vi "4 Bits Write.vi"(6 "E?E1:E2 (E1)":bool=TRUE, 9 "RS":bool, 10 "LCD data/cmd":u8 format="%.0x", 11 "device connection map":T1={"RS"="RS", "R/W"="RW", "E1"="E1", "E2"="E2", "DB4"="DB4", "DB5"="DB5", "DB6"="DB6", "DB7"="DB7"}) -> ()   [LabVIEW 2017, in "HD44780 FPGA.lvlib"]
uses:
  HD44780 FPGA.lvlib
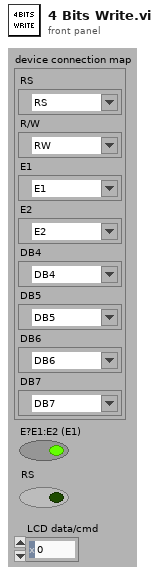
[diagram p1: front panel]
types:
  T1 = cluster{"RS":refnum<k21>, "R/W":refnum<k21>, "E1":refnum<k21>, "E2":refnum<k21>, "DB4":refnum<k21>, "DB5":refnum<k21>, "DB6":refnum<k21>, "DB7":refnum<k21>}
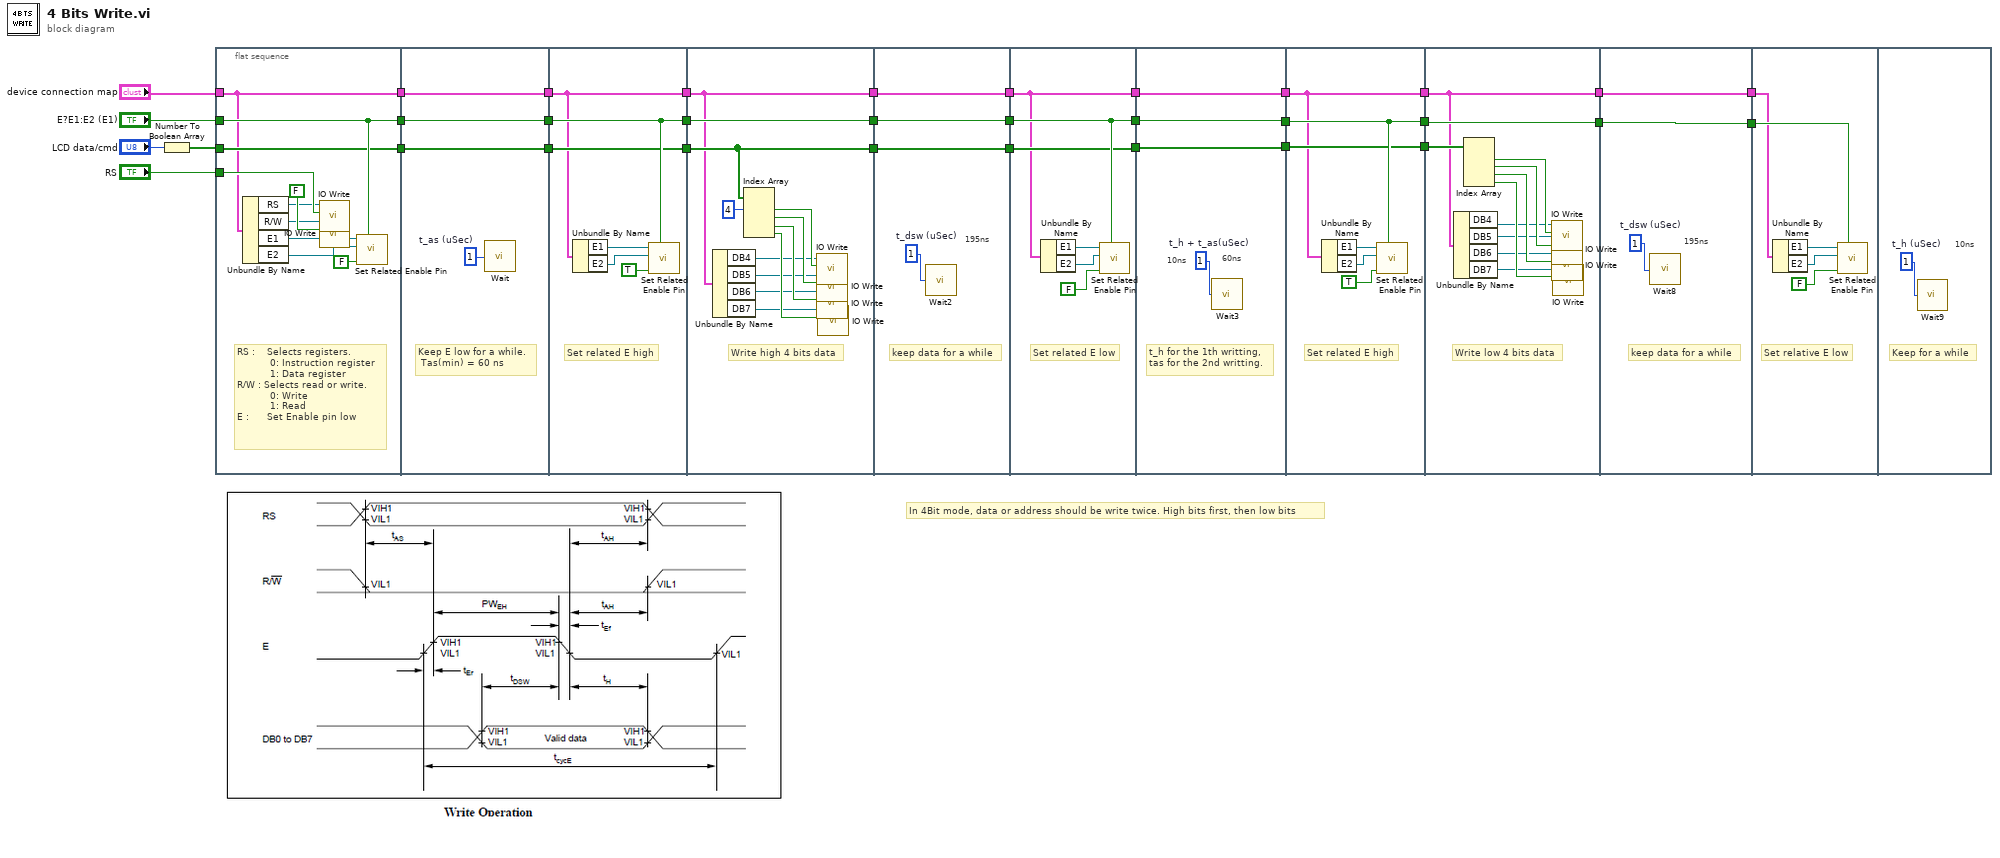
[diagram p0: block diagram]
diagram:
  # "In 4Bit mode, data or address should be write twice. High bits first, then low bits"
  n1 = Number To Boolean Array(number="LCD data/cmd") -> (Boolean array=w32:bool[])
  n2 = flat-sequence {
    tunnel: [w39] -> w29
    tunnel: [w40] -> w28
    tunnel: [w34] -> w11
    tunnel: w32 -> [w39]
    tunnel: "RS" -> [w43]
    tunnel: "E?E1:E2 (E1)" -> [w40]
    tunnel: "device connection map" -> [w34]
    tunnel: w29 -> [w46]
    tunnel: [w46] -> w27
    tunnel: w28 -> [w45]
    tunnel: [w45] -> w26
    tunnel: [w44] -> w12
    tunnel: w11 -> [w44]
    tunnel: w27 -> [w51]
    tunnel: [w51] -> w25
    tunnel: w26 -> [w52]
    tunnel: [w52] -> w24
    tunnel: [w48] -> w13
    tunnel: w12 -> [w48]
    tunnel: w25 -> [w64]
    tunnel: [w64] -> w23
    tunnel: w24 -> [w59]
    tunnel: [w59] -> w22
    tunnel: w13 -> [w54]
    tunnel: [w54] -> w8
    tunnel: w23 -> [w68]
    tunnel: [w68] -> w21
    tunnel: w22 -> [w67]
    tunnel: [w67] -> w20
    tunnel: [w66] -> w9
    tunnel: w8 -> [w66]
    tunnel: w21 -> [w73]
    tunnel: [w73] -> w19
    tunnel: w20 -> [w75]
    tunnel: [w75] -> w18
    tunnel: [w72] -> w10
    tunnel: w9 -> [w72]
    tunnel: w19 -> [w78]
    tunnel: [w78] -> w4
    tunnel: w18 -> [w77]
    tunnel: [w77] -> w3
    tunnel: w10 -> [w76]
    tunnel: [w76] -> w2
    tunnel: w4 -> [w83]
    tunnel: [w83] -> w17
    tunnel: w3 -> [w84]
    tunnel: [w84] -> w16
    tunnel: w2 -> [w80]
    tunnel: [w80] -> w7
    tunnel: w17 -> [w96]
    tunnel: w16 -> [w91]
    tunnel: [w91] -> w15
    tunnel: w7 -> [w86]
    tunnel: [w86] -> w6
    tunnel: w15 -> [w98]
    tunnel: [w98] -> w14
    tunnel: w6 -> [w97]
    tunnel: [w97] -> w5
    tunnel: w14 -> [w104]
    tunnel: w5 -> [w102]
    frame #0 {
      # "RS :    Selects registers.\n           0: Instruction register  \n           1: Data register\nR/W : Selects read or write.\n           0: Write\n           1: Read\nE :      Set Enable pin low"
      n3 = Unbundle By Name(w34) -> ("RS"=w38:refnum<k21>, "R/W"=w37:refnum<k21>, "E1"=w36:refnum<k21>, "E2"=w35:refnum<k21>)
      n4 = call "IO Write.vi"("data"=w43, "I/O"=w38) -> ()  [unwired: 10 in]
      n5 = call "IO Write.vi"("data"=FALSE, "I/O"=w37) -> ()  [unwired: 10 in]
      n6 = call "Set Related Enable Pin.vi"("E?E1:E2"=w40, "data"=FALSE, "E2"=w35, "E1"=w36) -> ()  [unwired: 8 in]
    }
    frame #1 {
      w47 = u32 1  # t_as (uSec)
      # "Keep E low for a while.\n Tas(min) = 60 ns"
      n7 = call "Wait"("Count(uSec)"=w47) -> ()  [unwired: 1 out]
    }
    frame #2 {
      # "Set related E high"
      n8 = Unbundle By Name(w48) -> ("E1"=w50:refnum<k21>, "E2"=w49:refnum<k21>)
      n9 = call "Set Related Enable Pin.vi"("E?E1:E2"=w52, "data"=TRUE, "E2"=w49, "E1"=w50) -> ()  [unwired: 8 in]
    }
    frame #3 {
      # "Write high 4 bits data"
      n10 = Unbundle By Name(w54) -> ("DB4"=w58:refnum<k21>, "DB5"=w57:refnum<k21>, "DB6"=w56:refnum<k21>, "DB7"=w55:refnum<k21>)
      n11 = Index Array(array=w64, index #1=4 ("index")) -> (element #1=w63:bool, element #2=w62:bool, element #3=w61:bool, element #4=w60:bool)  [unwired: 3 in]
      n12 = call "IO Write.vi"("data"=w63, "I/O"=w58) -> ()  [unwired: 10 in]
      n13 = call "IO Write.vi"("data"=w62, "I/O"=w57) -> ()  [unwired: 10 in]
      n14 = call "IO Write.vi"("data"=w61, "I/O"=w56) -> ()  [unwired: 10 in]
      n15 = call "IO Write.vi"("data"=w60, "I/O"=w55) -> ()  [unwired: 10 in]
    }
    frame #4 {
      w69 = u32 1  # t_dsw (uSec)
      # "keep data for a while"
      # "195ns"
      n16 = call "Wait2"("Count(uSec)"=w69) -> ()  [unwired: 1 out]
    }
    frame #5 {
      # "Set related E low"
      n17 = Unbundle By Name(w72) -> ("E1"=w71:refnum<k21>, "E2"=w70:refnum<k21>)
      n18 = call "Set Related Enable Pin.vi"("E?E1:E2"=w75, "data"=FALSE, "E2"=w70, "E1"=w71) -> ()  [unwired: 8 in]
    }
    frame #6 {
      w79 = u32 1  # t_h + t_as(uSec)
      # "60ns"
      # "t_h for the 1th writting, \ntas for the 2nd writting."
      # "10ns"
      n19 = call "Wait3"("Count(uSec)"=w79) -> ()  [unwired: 1 out]
    }
    frame #7 {
      # "Set related E high"
      n20 = Unbundle By Name(w80) -> ("E1"=w82:refnum<k21>, "E2"=w81:refnum<k21>)
      n21 = call "Set Related Enable Pin.vi"("E?E1:E2"=w84, "data"=TRUE, "E2"=w81, "E1"=w82) -> ()  [unwired: 8 in]
    }
    frame #8 {
      # "Write low 4 bits data"
      n22 = Unbundle By Name(w86) -> ("DB4"=w90:refnum<k21>, "DB5"=w89:refnum<k21>, "DB6"=w88:refnum<k21>, "DB7"=w87:refnum<k21>)
      n23 = Index Array(array=w96) -> (element #1=w95:bool, element #2=w94:bool, element #3=w93:bool, element #4=w92:bool)  [unwired: 4 in]
      n24 = call "IO Write.vi"("data"=w95, "I/O"=w90) -> ()  [unwired: 10 in]
      n25 = call "IO Write.vi"("data"=w94, "I/O"=w89) -> ()  [unwired: 10 in]
      n26 = call "IO Write.vi"("data"=w93, "I/O"=w88) -> ()  [unwired: 10 in]
      n27 = call "IO Write.vi"("data"=w92, "I/O"=w87) -> ()  [unwired: 10 in]
    }
    frame #9 {
      w99 = u32 1  # t_dsw (uSec)
      # "keep data for a while"
      # "195ns"
      n28 = call "Wait8"("Count(uSec)"=w99) -> ()  [unwired: 1 out]
    }
    frame #10 {
      # "Set relative E low"
      n29 = Unbundle By Name(w102) -> ("E1"=w101:refnum<k21>, "E2"=w100:refnum<k21>)
      n30 = call "Set Related Enable Pin.vi"("E?E1:E2"=w104, "data"=FALSE, "E2"=w100, "E1"=w101) -> ()  [unwired: 8 in]
    }
    frame #11 {
      w105 = u32 1  # t_h (uSec)
      # "Keep for a while"
      # "10ns"
      n31 = call "Wait9"("Count(uSec)"=w105) -> ()  [unwired: 1 out]
    }
  }
